vi "Ping Test.vi"() -> ()   [LabVIEW 2024]
doc: "Simple example that tests the Sift Ping service.\n\nRun this to verify that your credentials are valid."
uses:
  Sift API/Sift Client.lvclass
panel:
  out "Error":errorcluster
  out "Reponse":string
  in  "API Key":string
  in  "API URL":string
  # "Sift Ping Example"
  # "Instructions\n\n1. Fill in the API URL and API Key. Visit this URL for more information on authentication\n    https://docs.siftstack.com/docs/api/authentication\n\n2. Start the VI\n\n3. You should see a response from Sift."
  # "Run this example to verify connectivity to the API and credentials."
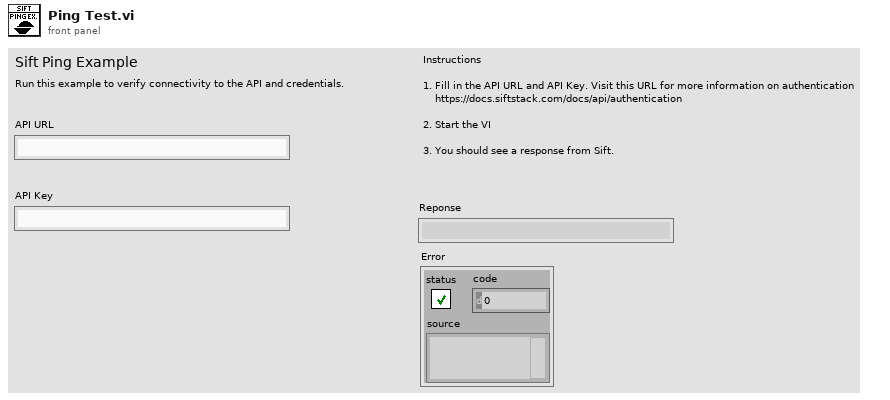
[diagram p1: front panel]
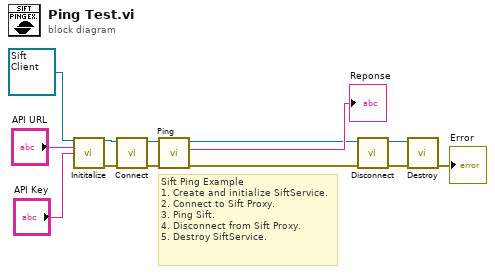
[diagram p0: block diagram]
diagram:
  # "Sift Ping Example\n1. Create and initialize SiftService.\n2. Connect to Sift Proxy.\n3. Ping Sift.\n4. Disconnect from Sift Proxy.\n5. Destroy SiftService."
  n1 = call-dynamic "Inititalize.vi"("Sift Client in"=refnum<class "Sift Client.lvclass"> refnum ("Sift Client.lvlib:Sift Client.lvclass"), "API URL"="API URL", "API Key"="API Key") -> ("Sift Client out"=w8:refnum<class "Sift Client.lvclass">, "error out"=w7:errorcluster)  [unwired: 11 in]
  n2 = call-dynamic "Connect.vi"("error in (no error)"=w7, "Sift Client in"=w8) -> ("error out"=w5:errorcluster, "Sift Client out"=w6:refnum<class "Sift Client.lvclass">)  [unwired: 7 in, 1 out]
  n3 = call-dynamic "Ping.vi"("error in (no error)"=w5, "Sift Client in"=w6) -> ("error out"=w3:errorcluster, "response"=→"Reponse":string, "Sift Client out"=w4:refnum<class "Sift Client.lvclass">)  [unwired: 7 in]
  n4 = call-dynamic "Disconnect.vi"("error in (no error)"=w3, "Sift Client in"=w4) -> ("error out"=w1:errorcluster, "Sift Client out"=w2:refnum<class "Sift Client.lvclass">)  [unwired: 8 in]
  n5 = call-dynamic "Destroy.vi"("error in (no error)"=w1, "Sift Client in"=w2) -> ("error out"=→"Error":errorcluster)  [unwired: 8 in, 1 out]
